vi "Save VI with XML Heaps.vi"(8 "error in (no error)":errorcluster, 9 "Heap Save Format (1:XML)":T1=1 items=["Off", "XML", "Binary", "Verbose Tagged Text", "Binary2"], 10 "VI Path (temporary file)":path=path "", 11 "VI Refnum In":refnum<vi>) -> (0 "error out":errorcluster, 2 "VI Path out":path, 3 "VI Refnum Out":refnum<vi>)   [LabVIEW 2026, in "VILab.lvlib"]
uses:
  VILab.lvlib
  CTLs/Heap Save Format.ctl
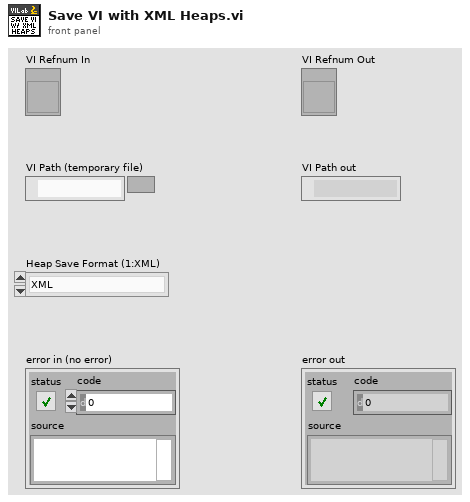
[diagram p1: front panel]
types:
  T1 = typedef "VILab.lvlib/Heap Save Format.ctl" = u16
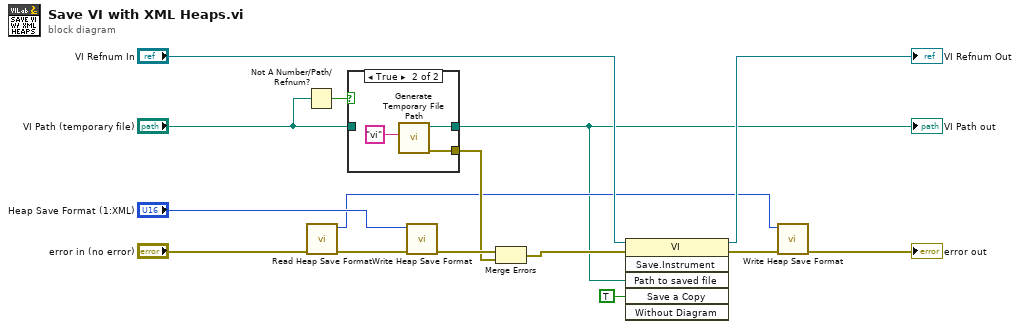
[diagram p0: block diagram]
diagram:
  n1 = Not A Number/Path/Refnum?(number/path/refnum="VI Path (temporary file)") -> (NaN/Path/Refnum?=w5:bool)
  n2 = call "Read Heap Save Format.vi"("error in (no error)"="error in (no error)") -> ("error out"=w13:errorcluster, "Heap Save Format"=w2:T1)  [unwired: 9 in]
  n3 = case shown="True" w5 {
    tunnel: [w16 w18] -> w1
    tunnel: "VI Path (temporary file)" -> [w16 _]
    tunnel: [_ w19] -> w10
    frame False {
    }
    frame True {
      n4 = call <vilib>:"Generate Temporary File Path.vi"("Temporary File Extension (tmp)"="vi") -> ("error out"=w19:errorcluster, "Unique Temporary File Path"=w18:path)  [unwired: 9 in]
    }
  }
  "VI Path out" <- w1
  n5 = call "Write Heap Save Format.vi"("error in (no error)"=w13, "Heap Save Format"="Heap Save Format (1:XML)") -> ("error out"=w11:errorcluster)  [unwired: 9 in]
  n6 = Merge Errors(w11, w10) -> (w9:errorcluster)
  n7 = invoke class="VI" method="Save.Instrument"(reference="VI Refnum In", error in=w9, "Path to saved file"=w1, "Save a Copy"=TRUE) -> (reference out=→"VI Refnum Out":refnum<vi>, error out=w12:errorcluster)  [unwired: 2 in, 4 out]
  n8 = call "Write Heap Save Format.vi"("error in (no error)"=w12, "Heap Save Format"=w2) -> ("error out"=→"error out":errorcluster)  [unwired: 9 in]
